vi "basic tester.vi"() -> ()   [LabVIEW 2015]
panel:
  out "counter":dbl
  in  "stop":bool
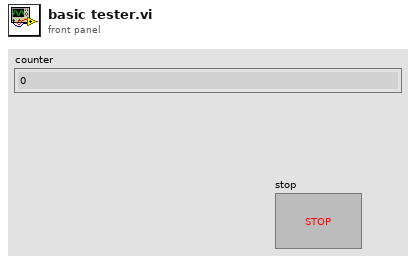
[diagram p1: front panel]
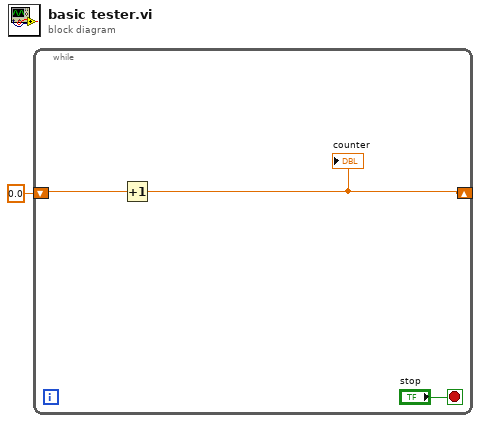
[diagram p0: block diagram]
diagram:
  n1 = while {
    shift-right: [w2] -> _
    shift-left: 0.0 -> [w3]
    stop <- "stop" stop-if-true
    n2 = Increment(x=w3) -> (x+1=w2:dbl)
    "counter" <- w2
  }
